vi "SentinelController v33.vi"() -> ()   [LabVIEW 2011] (continued)
                                tunnel: w513 -> [w608]
                                tunnel: w512 -> [w607]
                                frame #0 {
                                n2148 = while {
                                stop <- w517 continue-if-true
                                n2149 = local read "H1 Lock"() -> (w517:bool)
                                n2150 = Wait (ms)(milliseconds to wait=u32 1) -> ()  [unwired: 1 out]
                                }
                                }
                                frame #1 {
                                n2151 = local read "Program Parallelism"() -> (w521:u32)
                                n2152 = local read "H1 parallelism"() -> (w522:u32)
                                n2153 = Less?(x=w522, y=w521) -> (x < y?=w519:bool)
                                n2154 = local read "H1 allow lower parallelism"() -> (w520:bool)
                                n2155 = And(x=w519, y=w520) -> (x .and. y?=w518:bool)
                                n2156 = case shown="False" w518 {
                                tunnel: [w524 w535] -> w523
                                frame False {
                                n2157 = local read "VISA bus 1 resource name out hid"() -> (w532:refnum<visa-resource-name>)
                                n2158 = local read "Binning string from tester hid"() -> (w524:string)
                                n2159 = local read "VISA bus 1 error out hid"() -> (w533:errorcluster)
                                n2160 = local read "GPIB bus 1 traffic"() -> (w528:string)
                                n2161 = VISA Write(VISA resource name=w532, write buffer=w524, error in (no error)=w533) -> (VISA resource name out=w530:refnum<visa-resource-name>, error out=w531:errorcluster)  [unwired: 1 out]
                                n2162 = local write "VISA bus 1 resource name out hid"(w530) -> ()
                                n2163 = local write "VISA bus 1 error out hid"(w531) -> ()
                                n2164 = Unbundle By Name(w531) -> ("status"=w529:bool)
                                n2165 = Concatenate Strings(w528, "\r\n", "Bus 1 write: " ("string"), w524) -> (w526:string)
                                n2166 = local write "GPIB bus 1 write error"(w529) -> ()
                                n2167 = local write "GPIB bus 1 traffic"(w526) -> ()
                                }
                                frame True {
                                n2168 = local read "H1 parallelism"() -> (w534:u32)
                                n2169 = local read "Binning string from tester hid"() -> (w536:string)
                                n2170 = local read "VISA bus 1 resource name out hid"() -> (w547:refnum<visa-resource-name>)
                                n2171 = local read "VISA bus 1 error out hid"() -> (w548:errorcluster)
                                n2172 = Multiply(x=w534, y=u32 8) -> (x*y=w538:u32)
                                n2173 = local read "GPIB bus 1 traffic"() -> (w543:string)
                                n2174 = Decrement(x=w538) -> (x-1=w539:u32)
                                n2175 = String Subset(string=w536, length (rest)=w539) -> (substring=w535:string)  [unwired: 1 in]
                                n2176 = VISA Write(VISA resource name=w547, write buffer=w535, error in (no error)=w548) -> (VISA resource name out=w545:refnum<visa-resource-name>, error out=w546:errorcluster)  [unwired: 1 out]
                                n2177 = local write "VISA bus 1 resource name out hid"(w545) -> ()
                                n2178 = local write "VISA bus 1 error out hid"(w546) -> ()
                                n2179 = Unbundle By Name(w546) -> ("status"=w544:bool)
                                n2180 = Concatenate Strings(w543, "\r\n", "Bus 1 write: " ("string"), w535) -> (w541:string)
                                n2181 = local write "GPIB bus 1 traffic"(w541) -> ()
                                n2182 = local write "GPIB bus 1 write error"(w544) -> ()
                                }
                                }
                                }
                                frame #2 {
                                n2183 = local write "H1 Ready with sites"(FALSE ("waiting")) -> ()
                                n2184 = Tick Count (ms)() -> (millisecond timer value=w551:u32)
                                n2185 = Tick Count (ms)() -> (millisecond timer value=w552:u32)
                                n2186 = local write "H1 tt end hidden"(w551) -> ()
                                n2187 = local write "H1 it start hidden"(w552) -> ()
                                n2188 = local write "H1 Indexing"(TRUE ("waiting")) -> ()
                                n2189 = local write "H1 Testing"(FALSE ("waiting")) -> ()
                                }
                                frame #3 {
                                n2190 = local read "H1 tt start hidden"() -> (w561:u32)
                                n2191 = local read "H1 tt end hidden"() -> (w562:u32)
                                n2192 = while {
                                tunnel: [w580] -> w576 mode=indexing
                                shift-right: [w581] -> _
                                shift-left: w557 -> [w583]
                                stop <- w578 stop-if-true
                                n2193 = Match Pattern(string=w583, regular expression=" ") -> (before substring=w580:string, after substring=w581:string, offset past match=w579:i32)  [unwired: 2 out]
                                n2194 = Less Than 0?(x=w579) -> (x < 0?=w578:bool)
                                }
                                n2195 = Subtract(x=w562, y=w561) -> (x-y=w560:u32)
                                n2196 = Divide(x=w560, y=u32 1000) -> (x/y=w558:dbl)
                                n2197 = local write "H1 measured Test Time"(w558) -> ()
                                n2198 = Array Size(array=w576) -> (size(s)=w573:i32)
                                n2199 = Divide(x=w573, y=3) -> (x/y=w575:dbl)
                                n2200 = To Unsigned Byte Integer(number=w575) -> (unsigned 8bit integer=w571:u8)
                                n2201 = local read "H1 SITES? response hid"() -> (w568:string)
                                n2202 = local read "H1 parallelism"() -> (w567:u32)
                                n2203 = Not Equal?(x=w567, y=w571) -> (x != y?=w572:bool)
                                n2204 = for {
                                N: w571 -> [_]
                                tunnel: w576 -> [w606]
                                tunnel: w568 -> [w597]
                                shift-right: [w590] -> w555
                                shift-left: 0 -> [w589]
                                shift-right: [w586] -> w556
                                shift-left: 0 -> [w584]
                                i -> [w587]
                                n2205 = Increment(x=w584) -> (x+1=w585:i32)
                                n2206 = Increment(x=w589) -> (x+1=w588:i32)
                                n2207 = Increment(x=w587) -> (x+1=w605:i32)
                                n2208 = String Subset(string=w597, offset (0)=w587, length (rest)=1 ("length (rest)")) -> (substring=w593:string)
                                n2209 = Multiply(x=3, y=w605) -> (x*y=w599:i32)
                                n2210 = Equal?(x=w593, y="1") -> (x = y?=w591:bool)
                                n2211 = Decrement(x=w599) -> (x-1=w598:i32)
                                n2212 = Select(t=w588, s=w591, f=w589) -> (s? t:f=w590:i32)
                                n2213 = Index Array(array=w606, index=w598) -> (element=w603:string)
                                n2214 = Decimal String To Number(string=w603, offset=0) -> (number=w601:i32)  [unwired: 1 in, 1 out]
                                n2215 = Equal?(x=w601, y=1) -> (x = y?=w594:bool)
                                n2216 = And(x=w594, y=w591) -> (x .and. y?=w595:bool)
                                n2217 = Select(t=w585, s=w595, f=w584) -> (s? t:f=w586:i32)
                                }
                                n2218 = case shown="True" w572 {
                                frame False {
                                }
                                frame True {
                                n2219 = One Button Dialog(message="Warning:\nH1 Parallelism Mismatch!\nEither allow this from the system configuration tab\nor change the parallelism on H2. This message will\ncontinue until the problem is corrected.") -> ()  [unwired: 1 in, 1 out]
                                }
                                }
                                n2220 = local read "H1 Device Count"() -> (w564:u32)
                                n2221 = local read "H1 Good Units"() -> (w565:u32)
                                n2222 = Add(x=w565, y=w556) -> (x+y=w566:u32)
                                n2223 = Add(x=w564, y=w555) -> (x+y=w563:u32)
                                n2224 = local write "H1 Good Units"(w566) -> ()
                                n2225 = local write "H1 Device Count"(w563) -> ()
                                }
                                frame #4 {
                                n2226 = local read "H1 Device Count"() -> (w612:u32)
                                n2227 = Divide(x=w608, y=w607) -> (x/y=w609:dbl)
                                n2228 = local read "H1 Good Units"() -> (w613:u32)
                                n2229 = Multiply(x=w609, y=100.0) -> (x*y=w611:dbl)
                                n2230 = Divide(x=w613, y=w612) -> (x/y=w616:dbl)
                                n2231 = local write "H1 cycle yield hid"(w611) -> ()
                                n2232 = Multiply(x=w616, y=100.0) -> (x*y=w614:dbl)
                                n2233 = local write "H1 lot yield mon"(w614) -> ()
                                }
                                frame #5 {
                                n2234 = local read "H1 online"() -> (w617:bool)
                                n2235 = local read "POWER"() -> (w618:bool)
                                n2236 = Compound Arithmetic op=AND(w617, w618) -> (w619:bool)
                                n2237 = case shown="True" w619 {
                                frame False {
                                n2238 = local write "MT99XX tester states H1 hid"(SC_MT99XX_tester_states."closing bus" ("SC virtual tester states")) -> ()
                                }
                                frame True {
                                n2239 = local write "MT99XX tester states H1 hid"(SC_MT99XX_tester_states."polling *SITES?" ("SC virtual tester states")) -> ()
                                }
                                }
                                }
                                }
                                }
                                frame "closing bus" {
                                n2240 = local read "GPIB bus 1 traffic"() -> (w626:string)
                                n2241 = local write "Exit SC tester H1 StMach hid"(TRUE ("Exit H1 state machine hid")) -> ()
                                n2242 = local read "VISA bus 1 resource name out hid"() -> (w630:refnum<visa-resource-name>)
                                n2243 = local read "VISA bus 1 error out hid"() -> (w629:errorcluster)
                                n2244 = Concatenate Strings(w626, "\r\n", "Bus 1: closing " ("string")) -> (w624:string)
                                n2245 = local write "GPIB bus 1 traffic"(w624) -> ()
                                n2246 = VISA Close(VISA resource name=w630, error in (no error)=w629) -> (error out=w628:errorcluster)
                                n2247 = Unbundle By Name(w628) -> ("status"=w627:bool)
                                n2248 = local write "VISA bus 1 close error"(w627) -> ()
                                }
                              }
                            }
                            frame #1 {
                              n2249 = local read "Slow for  Diagnostics"() -> (w631:bool)
                              n2250 = case shown="False" w631 {
                                frame False {
                                }
                                frame True {
                                n2251 = local read "GPIB wait time (ms)"() -> (w632:u32)
                                n2252 = Wait (ms)(milliseconds to wait=w632) -> ()  [unwired: 1 out]
                                }
                              }
                            }
                          }
                        }
                        frame "DeltaDesign" {
                          n2253 = local write "MT99XX tester states H1 hid"(SC_MT99XX_tester_states."initializing bus" ("SC virtual tester states")) -> ()
                          n2254 = flat-sequence {
                            frame #0 {
                              n2255 = local read "MT99XX tester states H1 hid"() -> (w634:T4)
                              n2256 = case shown="\"binning\"" w634 {
                                frame "initializing bus", Default {
                                n2257 = flat-sequence {
                                frame #0 {
                                # "bus 1"
                                n2258 = local read "GPIB wait timeout hid"() -> (w638:u32)
                                n2259 = local read "SentCtrl talks to handler 1 at"() -> (w639:refnum<visa-resource-name>)
                                n2260 = local read "GPIB wait timeout hid"() -> (w637:u32)
                                n2261 = VISA Open(timeout (0)=w638, VISA resource name=w639) -> (VISA resource name=w636:refnum<visa-resource-name>, error out=w641:errorcluster)  [unwired: 3 in]
                                n2262 = property class="GPIB Instr"(reference=w636, error in=w641, "Timeout"=w637) -> (error out=w635:errorcluster)  [unwired: 1 out]
                                n2263 = local write "VISA bus 1 resource name out hid"(w636) -> ()
                                n2264 = Unbundle By Name(w635) -> ("status"=w640:bool)
                                n2265 = local write "VISA bus 1 open error"(w640) -> ()
                                n2266 = local write "VISA bus 1 error out hid"(w635) -> ()
                                }
                                frame #1 {
                                n2267 = local write "Exit SC tester H1 StMach hid"(FALSE ("Exit H1 state machine hid")) -> ()
                                n2268 = Concatenate Strings("Bus 1 initializing" ("string"), "\r\n") -> (w644:string)
                                n2269 = local write "GPIB bus 1 traffic"(w644) -> ()
                                }
                                frame #2 {
                                n2270 = local write "MT99XX tester states H1 hid"(SC_MT99XX_tester_states."sending *IDN?" ("SC virtual tester states")) -> ()
                                }
                                }
                                }
                                frame "sending *IDN?" {
                                n2271 = flat-sequence {
                                tunnel: [w656] -> w649
                                tunnel: [w655] -> w648
                                tunnel: w649 -> [w670]
                                tunnel: w648 -> [w669]
                                tunnel: [w660] -> w647
                                tunnel: w647 -> [w671]
                                frame #0 {
                                w650 = "*IDN?"
                                n2272 = local read "VISA bus 1 resource name out hid"() -> (w659:refnum<visa-resource-name>)
                                n2273 = local read "GPIB bus 1 traffic"() -> (w654:string)
                                n2274 = local read "VISA bus 1 error out hid"() -> (w658:errorcluster)
                                n2275 = Concatenate Strings(w654, "\r\n", "Bus 1 write: " ("string"), w650) -> (w652:string)
                                n2276 = VISA Write(VISA resource name=w659, write buffer=w650, error in (no error)=w658) -> (VISA resource name out=w656:refnum<visa-resource-name>, error out=w655:errorcluster)  [unwired: 1 out]
                                n2277 = Unbundle By Name(w655) -> ("status"=w657:bool)
                                n2278 = local write "GPIB bus 1 traffic"(w652) -> ()
                                n2279 = local write "GPIB bus 1 write error"(w657) -> ()
                                }
                                frame #1 {
                                n2280 = local read "GPIB bus 1 traffic"() -> (w662:string)
                                n2281 = VISA Read(VISA resource name=w670, byte count=u32 256, error in (no error)=w669) -> (VISA resource name out=w667:refnum<visa-resource-name>, read buffer=w661:string, error out=w666:errorcluster)  [unwired: 1 out]
                                n2282 = local write "VISA bus 1 resource name out hid"(w667) -> ()
                                n2283 = Unbundle By Name(w666) -> ("status"=w660:bool)
                                n2284 = local write "H1 response to *IDN? hid"(w661) -> ()
                                n2285 = local write "GPIB bus 1 read error"(w660) -> ()
                                n2286 = Concatenate Strings(w662, "\r\n", "Bus 1 read: " ("string"), w661) -> (w664:string)
                                n2287 = local write "GPIB bus 1 traffic"(w664) -> ()
                                }
                                frame #2 {
                                n2288 = case shown="False" w671 {
                                frame False {
                                n2289 = local write "MT99XX tester states H1 hid"(SC_MT99XX_tester_states."polling *SITES?" ("SC virtual tester states")) -> ()
                                }
                                frame True {
                                n2290 = flat-sequence {
                                frame #0 {
                                n2291 = while {
                                stop <- w674 stop-if-true
                                n2292 = One Button Dialog(message="Warning:\nVirtual tester does not get a response\nto *IDN? from handler 1.\nCheck GPIB cable and that  handler 1 \nis running and ready to issue a start of test\nby responding with sites ready.", button name ("OK")="Dismiss and retry") -> (true=w674:bool)
                                n2293 = Wait (ms)(milliseconds to wait=u32 100) -> ()  [unwired: 1 out]
                                }
                                }
                                frame #1 {
                                n2294 = local write "H1 online"(FALSE ("H1 online")) -> ()
                                }
                                frame #2 {
                                n2295 = local write "MT99XX tester states H1 hid"(SC_MT99XX_tester_states."sending *IDN?" ("SC virtual tester states")) -> ()
                                }
                                }
                                }
                                }
                                }
                                }
                                }
                                frame "polling *SITES?" {
                                n2296 = flat-sequence {
                                tunnel: [w682] -> w680
                                tunnel: [w681] -> w679
                                tunnel: w680 -> [w718]
                                tunnel: w679 -> [w717]
                                frame #0 {
                                n2297 = while {
                                tunnel: [w686] -> w682
                                tunnel: [w684] -> w681
                                stop <- w683 stop-if-true
                                n2298 = stacked-sequence {
                                tunnel: [w698] -> w688
                                tunnel: [w697] -> w687
                                frame #0 {
                                w690 = "*SITES?"
                                n2299 = local read "VISA bus 1 resource name out hid"() -> (w696:refnum<visa-resource-name>)
                                n2300 = local read "VISA bus 1 error out hid"() -> (w695:errorcluster)
                                n2301 = Concatenate Strings("Handler 1 cycle start" ("string"), "\r\n", "Bus 1 write: " ("string"), w690) -> (w692:string)
                                n2302 = VISA Write(VISA resource name=w696, write buffer=w690, error in (no error)=w695) -> (VISA resource name out=w698:refnum<visa-resource-name>, error out=w697:errorcluster)  [unwired: 1 out]
                                n2303 = Unbundle By Name(w697) -> ("status"=w694:bool)
                                n2304 = local write "GPIB bus 1 traffic"(w692) -> ()
                                n2305 = local write "GPIB bus 1 write error"(w694) -> ()
                                }
                                }
                                n2306 = Wait (ms)(milliseconds to wait=u32 1) -> ()  [unwired: 1 out]
                                n2307 = flat-sequence {
                                tunnel: w688 -> [w716]
                                tunnel: w687 -> [w715]
                                tunnel: [w703] -> w686
                                tunnel: [w699] -> w684
                                tunnel: [w700] -> w683
                                frame #0 {
                                n2308 = local read "GPIB bus 1 traffic"() -> (w708:string)
                                n2309 = VISA Read(VISA resource name=w716, byte count=u32 256, error in (no error)=w715) -> (read buffer=w703:string, error out=w702:errorcluster)  [unwired: 2 out]
                                n2310 = Unbundle By Name(w702) -> ("status"=w699:bool)
                                n2311 = String Length(string=w703) -> (length=w705:i32)
                                n2312 = Scan Value(string=w703, format string="%b", default (0 dbl)=u8 0) -> (value=w707:u8)  [unwired: 1 out]
                                n2313 = Concatenate Strings(w708, "\r\n", "Bus 1 read: " ("string"), w703) -> (w710:string)
                                n2314 = local write "GPIB bus 1 read error"(w699) -> ()
                                n2315 = Greater Than 0?(x=w705) -> (x > 0?=w704:bool)
                                n2316 = Greater Than 0?(x=w707) -> (x > 0?=w706:bool)
                                n2317 = local write "GPIB bus 1 traffic"(w710) -> ()
                                n2318 = And(x=w704, y=w706) -> (x .and. y?=w701:bool)
                                n2319 = Or(x=w701, y=w699) -> (x .or. y?=w700:bool)
                                }
                                }
                                }
                                }
                                frame #1 {
                                n2320 = case shown="False" w717 {
                                tunnel: w718 -> [w719 _]
                                frame False {
                                n2321 = flat-sequence {
                                tunnel: w719 -> [w720]
                                frame #0 {
                                n2322 = String Length(string=w720) -> (length=w721:i32)
                                n2323 = local write "H1 SITES? response hid"(w720) -> ()
                                n2324 = local write "H1 parallelism"(w721) -> ()
                                }
                                frame #1 {
                                # "This block adds zeroes (sites not ready)\nto SITES READY from handlers when the\nhandler is running at a lower parallelism\nthan the test program, but has the same\npin mapping for the active sites in common."
                                n2325 = local read "Program Parallelism"() -> (w725:u32)
                                n2326 = local read "H1 allow lower parallelism"() -> (w724:bool)
                                n2327 = local read "H1 parallelism"() -> (w726:u32)
                                n2328 = Less?(x=w726, y=w725) -> (x < y?=w723:bool)
                                n2329 = And(x=w723, y=w724) -> (x .and. y?=w722:bool)
                                n2330 = case shown="True" w722 {
                                frame False {
                                n2331 = local read "Program Parallelism"() -> (w729:u32)
                                n2332 = local read "H1 parallelism"() -> (w727:u32)
                                n2333 = Greater?(x=w727, y=w729) -> (0:w728:bool)
                                n2334 = case shown="True" w728 {
                                frame False {
                                # "parallelisms must match if arriving here"
                                n2335 = local write "MT99XX tester states H1 hid"(SC_MT99XX_tester_states."testing" ("SC virtual tester states")) -> ()
                                }
                                frame True {
                                n2336 = local write "MT99XX tester states H1 hid"(SC_MT99XX_tester_states."closing bus" ("SC virtual tester states")) -> ()
                                n2337 = local write "POWER"(FALSE ("POWER")) -> ()
                                n2338 = One Button Dialog(message="Fatal error 300:\nTest program cannot support higher\nparallelism on handler 1.\nThe Sentinel Controller program is shutting down.\nPlease correct the mismatch and restart.") -> ()  [unwired: 1 in, 1 out]
                                }
                                }
                                }
                                frame True {
                                n2339 = local read "Program Parallelism"() -> (w739:u32)
                                n2340 = local read "H1 parallelism"() -> (w736:u32)
                                n2341 = local read "H1 SITES? response hid"() -> (w737:string)
                                n2342 = Subtract(x=w739, y=w736) -> (x-y=w738:u32)
                                n2343 = for {
                                N: w738 -> [_]
                                shift-right: [w740] -> w734
                                shift-left: w737 -> [w741]
                                n2344 = Concatenate Strings(w741, "0" ("string")) -> (w740:string)
                                }
                                n2345 = local write "H1 SITES? response hid"(w734) -> ()
                                n2346 = local write "MT99XX tester states H1 hid"(SC_MT99XX_tester_states."testing" ("SC virtual tester states")) -> ()
                                }
                                }
                                }
                                frame #2 {
                                n2347 = Tick Count (ms)() -> (millisecond timer value=w747:u32)
                                n2348 = Tick Count (ms)() -> (millisecond timer value=w746:u32)
                                n2349 = local write "H1 Ready with sites"(TRUE ("H2 Waiting")) -> ()
                                n2350 = local write "H1 wt start hidden"(w747) -> ()
                                n2351 = local write "H1 it end hidden"(w746) -> ()
                                n2352 = local write "H1 Indexing"(FALSE ("h1 indexing")) -> ()
                                n2353 = local write "H1 Testing"(FALSE ("h1 indexing")) -> ()
                                }
                                frame #3 {
                                n2354 = local read "H1 it start hidden"() -> (w751:u32)
                                n2355 = local read "H1 it end hidden"() -> (w752:u32)
                                n2356 = Subtract(x=w752, y=w751) -> (x-y=w748:u32)
                                n2357 = Divide(x=w748, y=u32 1000) -> (x/y=w750:dbl)
                                n2358 = local write "MT99XX tester states H1 hid"(SC_MT99XX_tester_states."testing" ("SC virtual tester states")) -> ()
                                n2359 = local write "H1 measured Index Time"(w750) -> ()
                                }
                                }
                                }
                                frame True {
                                n2360 = flat-sequence {
                                frame #0 {
                                n2361 = local read "VISA bus 1 resource name out hid"() -> (w756:refnum<visa-resource-name>)
                                n2362 = local read "VISA bus 1 error out hid"() -> (w757:errorcluster)
                                n2363 = VISA Close(VISA resource name=w756, error in (no error)=w757) -> (error out=w755:errorcluster)
                                n2364 = Unbundle By Name(w755) -> ("status"=w754:bool)
                                n2365 = local write "VISA bus 1 close error"(w754) -> ()
                                }
                                frame #1 {
                                n2366 = local write "VISA bus 1 close error"(FALSE ("VISA bus 1 close error")) -> ()
                                n2367 = Concatenate Strings("Bus 1 error  while reading,\nclosing Bus 1 and re-initializing" ("string"), "\r\n") -> (w760:string)
                                n2368 = local write "GPIB bus 1 traffic"(w760) -> ()
                                }
                                frame #2 {
                                n2369 = local write "MT99XX tester states H1 hid"(SC_MT99XX_tester_states."initializing bus" ("SC virtual tester states")) -> ()
                                }
                                }
                                }
                                }
                                }
                                }
                                }
                                frame "testing" {
                                n2370 = flat-sequence {
                                frame #0 {
                                n2371 = while {
                                stop <- w763 stop-if-true
                                n2372 = local read "H1 Lock"() -> (w763:bool)
                                n2373 = Wait (ms)(milliseconds to wait=u32 1) -> ()  [unwired: 1 out]
                                }
                                }
                                frame #1 {
                                n2374 = Tick Count (ms)() -> (millisecond timer value=w774:u32)
                                n2375 = Tick Count (ms)() -> (millisecond timer value=w773:u32)
                                n2376 = local write "H1 Testing"(TRUE ("testing")) -> ()
                                n2377 = local write "H1 Ready with sites"(FALSE ("H1 Waiting")) -> ()
                                n2378 = local write "H1 Indexing"(FALSE ("waiting")) -> ()
                                n2379 = local write "H1 wt end hidden"(w774) -> ()
                                n2380 = local write "H1 tt start hidden"(w773) -> ()
                                n2381 = local read "GPIB bus 1 traffic"() -> (w766:string)
                                n2382 = Concatenate Strings(w766, "\r\n", "Bus 1: " ("string"), "testing" ("string")) -> (w768:string)
                                n2383 = local write "GPIB bus 1 traffic"(w768) -> ()
                                }
                                frame #2 {
                                n2384 = local read "H1 wt start hidden"() -> (w778:u32)
                                n2385 = local read "H1 wt end hidden"() -> (w779:u32)
                                n2386 = Subtract(x=w779, y=w778) -> (x-y=w777:u32)
                                n2387 = Divide(x=w777, y=u32 1000) -> (x/y=w775:dbl)
                                n2388 = local write "H1 measured Wait Time"(w775) -> ()
                                }
                                frame #3 {
                                n2389 = local write "MT99XX tester states H1 hid"(SC_MT99XX_tester_states."binning" ("SC virtual tester states")) -> ()
                                }
                                }
                                }
                                frame "binning" {
                                n2390 = flat-sequence {
                                tunnel: [w792] -> w784
                                tunnel: [w819] -> w783
                                tunnel: w784 -> [w819]
                                tunnel: w783 -> [w826]
                                tunnel: [w825] -> w782
                                tunnel: [w824] -> w781
                                tunnel: w782 -> [w877]
                                tunnel: w781 -> [w876]
                                frame #0 {
                                n2391 = while {
                                stop <- w786 continue-if-true
                                n2392 = local read "H1 Lock"() -> (w786:bool)
                                n2393 = Wait (ms)(milliseconds to wait=u32 1) -> ()  [unwired: 1 out]
                                }
                                }
                                frame #1 {
                                n2394 = local read "Program Parallelism"() -> (w790:u32)
                                n2395 = local read "H1 parallelism"() -> (w791:u32)
                                n2396 = Less?(x=w791, y=w790) -> (x < y?=w788:bool)
                                n2397 = local read "H1 allow lower parallelism"() -> (w789:bool)
                                n2398 = And(x=w788, y=w789) -> (x .and. y?=w787:bool)
                                n2399 = case shown="False" w787 {
                                tunnel: [w793 w804] -> w792
                                frame False {
                                n2400 = local read "VISA bus 1 resource name out hid"() -> (w801:refnum<visa-resource-name>)
                                n2401 = local read "Binning string from tester hid"() -> (w793:string)
                                n2402 = local read "VISA bus 1 error out hid"() -> (w802:errorcluster)
                                n2403 = local read "GPIB bus 1 traffic"() -> (w797:string)
                                n2404 = VISA Write(VISA resource name=w801, write buffer=w793, error in (no error)=w802) -> (VISA resource name out=w799:refnum<visa-resource-name>, error out=w800:errorcluster)  [unwired: 1 out]
                                n2405 = local write "VISA bus 1 resource name out hid"(w799) -> ()
                                n2406 = local write "VISA bus 1 error out hid"(w800) -> ()
                                n2407 = Unbundle By Name(w800) -> ("status"=w798:bool)
                                n2408 = Concatenate Strings(w797, "\r\n", "Bus 1 write: " ("string"), w793) -> (w795:string)
                                n2409 = local write "GPIB bus 1 write error"(w798) -> ()
                                n2410 = local write "GPIB bus 1 traffic"(w795) -> ()
                                }
                                frame True {
                                n2411 = local read "H1 parallelism"() -> (w803:u32)
                                n2412 = local read "Binning string from tester hid"() -> (w805:string)
                                n2413 = local read "VISA bus 1 resource name out hid"() -> (w816:refnum<visa-resource-name>)
                                n2414 = local read "VISA bus 1 error out hid"() -> (w817:errorcluster)
                                n2415 = Multiply(x=w803, y=u32 8) -> (x*y=w807:u32)
                                n2416 = local read "GPIB bus 1 traffic"() -> (w812:string)
                                n2417 = Decrement(x=w807) -> (x-1=w808:u32)
                                n2418 = String Subset(string=w805, length (rest)=w808) -> (substring=w804:string)  [unwired: 1 in]
                                n2419 = VISA Write(VISA resource name=w816, write buffer=w804, error in (no error)=w817) -> (VISA resource name out=w814:refnum<visa-resource-name>, error out=w815:errorcluster)  [unwired: 1 out]
                                n2420 = local write "VISA bus 1 resource name out hid"(w814) -> ()
                                n2421 = local write "VISA bus 1 error out hid"(w815) -> ()
                                n2422 = Unbundle By Name(w815) -> ("status"=w813:bool)
                                n2423 = Concatenate Strings(w812, "\r\n", "Bus 1 write: " ("string"), w804) -> (w810:string)
                                n2424 = local write "GPIB bus 1 traffic"(w810) -> ()
                                n2425 = local write "GPIB bus 1 write error"(w813) -> ()
                                }
                                }
                                }
                                frame #2 {
                                n2426 = local write "H1 Ready with sites"(FALSE ("waiting")) -> ()
                                n2427 = Tick Count (ms)() -> (millisecond timer value=w820:u32)
                                n2428 = Tick Count (ms)() -> (millisecond timer value=w821:u32)
                                n2429 = local write "H1 tt end hidden"(w820) -> ()
                                n2430 = local write "H1 it start hidden"(w821) -> ()
                                n2431 = local write "H1 Indexing"(TRUE ("waiting")) -> ()
                                n2432 = local write "H1 Testing"(FALSE ("waiting")) -> ()
                                }
                                frame #3 {
                                n2433 = local read "H1 tt start hidden"() -> (w830:u32)
                                n2434 = while {
                                tunnel: [w849] -> w845 mode=indexing
                                shift-right: [w850] -> _
                                shift-left: w826 -> [w852]
                                stop <- w847 stop-if-true
                                n2435 = Match Pattern(string=w852, regular expression=" ") -> (before substring=w849:string, after substring=w850:string, offset past match=w848:i32)  [unwired: 2 out]
                                n2436 = Less Than 0?(x=w848) -> (x < 0?=w847:bool)
                                }
                                n2437 = local read "H1 tt end hidden"() -> (w831:u32)
                                n2438 = Subtract(x=w831, y=w830) -> (x-y=w829:u32)
                                n2439 = Divide(x=w829, y=u32 1000) -> (x/y=w827:dbl)
                                n2440 = local write "H1 measured Test Time"(w827) -> ()
                                n2441 = Array Size(array=w845) -> (size(s)=w842:i32)
                                n2442 = Divide(x=w842, y=3) -> (x/y=w844:dbl)
                                n2443 = To Unsigned Byte Integer(number=w844) -> (unsigned 8bit integer=w840:u8)
                                n2444 = local read "H1 SITES? response hid"() -> (w837:string)
                                n2445 = local read "H1 parallelism"() -> (w836:u32)
                                n2446 = Not Equal?(x=w836, y=w840) -> (x != y?=w841:bool)
                                n2447 = for {
                                N: w840 -> [_]
                                tunnel: w845 -> [w875]
                                tunnel: w837 -> [w866]
                                shift-right: [w859] -> w824
                                shift-left: 0 -> [w858]
                                shift-right: [w855] -> w825
                                shift-left: 0 -> [w853]
                                i -> [w856]
                                n2448 = Increment(x=w853) -> (x+1=w854:i32)
                                n2449 = Increment(x=w858) -> (x+1=w857:i32)
                                n2450 = Increment(x=w856) -> (x+1=w874:i32)
                                n2451 = String Subset(string=w866, offset (0)=w856, length (rest)=1 ("length (rest)")) -> (substring=w862:string)
                                n2452 = Multiply(x=3, y=w874) -> (x*y=w868:i32)
                                n2453 = Equal?(x=w862, y="1") -> (x = y?=w860:bool)
                                n2454 = Decrement(x=w868) -> (x-1=w867:i32)
                                n2455 = Select(t=w857, s=w860, f=w858) -> (s? t:f=w859:i32)
                                n2456 = Index Array(array=w875, index=w867) -> (element=w872:string)
                                n2457 = Decimal String To Number(string=w872, offset=0) -> (number=w870:i32)  [unwired: 1 in, 1 out]
                                n2458 = Equal?(x=w870, y=1) -> (x = y?=w863:bool)
                                n2459 = And(x=w863, y=w860) -> (x .and. y?=w864:bool)
                                n2460 = Select(t=w854, s=w864, f=w853) -> (s? t:f=w855:i32)
                                }
                                n2461 = case shown="True" w841 {
                                frame False {
                                }
                                frame True {
                                n2462 = One Button Dialog(message="Warning:\nH1 Parallelism Mismatch!\nEither allow this from the system configuration tab\nor change the parallelism on H2. This message will\ncontinue until the problem is corrected.") -> ()  [unwired: 1 in, 1 out]
                                }
                                }
                                n2463 = local read "H1 Device Count"() -> (w833:u32)
                                n2464 = local read "H1 Good Units"() -> (w834:u32)
                                n2465 = Add(x=w834, y=w825) -> (x+y=w835:u32)
                                n2466 = Add(x=w833, y=w824) -> (x+y=w832:u32)
                                n2467 = local write "H1 Good Units"(w835) -> ()
                                n2468 = local write "H1 Device Count"(w832) -> ()
                                }
                                frame #4 {
                                n2469 = local read "H1 Device Count"() -> (w881:u32)
                                n2470 = Divide(x=w877, y=w876) -> (x/y=w878:dbl)
                                n2471 = local read "H1 Good Units"() -> (w882:u32)
                                n2472 = Multiply(x=w878, y=100.0) -> (x*y=w880:dbl)
                                n2473 = Divide(x=w882, y=w881) -> (x/y=w885:dbl)
                                n2474 = local write "H1 cycle yield hid"(w880) -> ()
                                n2475 = Multiply(x=w885, y=100.0) -> (x*y=w883:dbl)
                                n2476 = local write "H1 lot yield mon"(w883) -> ()
                                }
                                frame #5 {
                                n2477 = local read "H1 online"() -> (w886:bool)
                                n2478 = local read "POWER"() -> (w887:bool)
                                n2479 = Compound Arithmetic op=AND(w886, w887) -> (w888:bool)
                                n2480 = case shown="True" w888 {
                                frame False {
                                n2481 = local write "MT99XX tester states H1 hid"(SC_MT99XX_tester_states."closing bus" ("SC virtual tester states")) -> ()
                                }
                                frame True {
                                n2482 = local write "MT99XX tester states H1 hid"(SC_MT99XX_tester_states."polling *SITES?" ("SC virtual tester states")) -> ()
                                }
                                }
                                }
                                }
                                }
                                frame "closing bus" {
                                n2483 = local read "GPIB bus 1 traffic"() -> (w895:string)
                                n2484 = local write "Exit SC tester H1 StMach hid"(TRUE ("Exit H1 state machine hid")) -> ()
                                n2485 = local read "VISA bus 1 resource name out hid"() -> (w899:refnum<visa-resource-name>)
                                n2486 = local read "VISA bus 1 error out hid"() -> (w898:errorcluster)
                                n2487 = Concatenate Strings(w895, "\r\n", "Bus 1: closing " ("string")) -> (w893:string)
                                n2488 = local write "GPIB bus 1 traffic"(w893) -> ()
                                n2489 = VISA Close(VISA resource name=w899, error in (no error)=w898) -> (error out=w897:errorcluster)
                                n2490 = Unbundle By Name(w897) -> ("status"=w896:bool)
                                n2491 = local write "VISA bus 1 close error"(w896) -> ()
                                }
                              }
                            }
                            frame #1 {
                              n2492 = local read "Slow for  Diagnostics"() -> (w900:bool)
                              n2493 = case shown="False" w900 {
                                frame False {
                                }
                                frame True {
                                n2494 = local read "GPIB wait time (ms)"() -> (w901:u32)
                                n2495 = Wait (ms)(milliseconds to wait=w901) -> ()  [unwired: 1 out]
                                }
                              }
                            }
                          }
                        }
                        frame "Seiko-Epson NS6040" {
                          n2496 = local write "NS6040 tester states H1 hid"(SC_NS6040_tester_states."initializing bus" ("NS6040 tester states H1 hid")) -> ()
                          n2497 = while {
                            stop <- w903 stop-if-true
                            n2498 = flat-sequence {
                              frame #0 {
                                n2499 = local read "NS6040 tester states H1 hid"() -> (w904:T3)
                                n2500 = case shown="\"testing\"" w904 {
                                frame "initializing bus", Default {
                                n2501 = flat-sequence {
                                frame #0 {
                                # "bus 1"
                                n2502 = local read "GPIB wait timeout hid"() -> (w908:u32)
                                n2503 = local read "SentCtrl talks to handler 1 at"() -> (w909:refnum<visa-resource-name>)
                                n2504 = local read "GPIB wait timeout hid"() -> (w907:u32)
                                n2505 = VISA Open(timeout (0)=w908, VISA resource name=w909) -> (VISA resource name=w906:refnum<visa-resource-name>, error out=w911:errorcluster)  [unwired: 3 in]
                                n2506 = property class="GPIB Instr"(reference=w906, error in=w911, "Timeout"=w907) -> (error out=w905:errorcluster)  [unwired: 1 out]
                                n2507 = local write "VISA bus 1 resource name out hid"(w906) -> ()
                                n2508 = Unbundle By Name(w905) -> ("status"=w910:bool)
                                n2509 = local write "VISA bus 1 open error"(w910) -> ()
                                n2510 = local write "VISA bus 1 error out hid"(w905) -> ()
                                }
                                frame #1 {
                                n2511 = local write "Exit SC tester H1 StMach hid"(FALSE ("Exit H1 state machine hid")) -> ()
                                n2512 = Concatenate Strings("Bus 1 initializing" ("string"), "\r\n") -> (w914:string)
                                n2513 = local write "GPIB bus 1 traffic"(w914) -> ()
                                }
                                frame #2 {
                                n2514 = local write "NS6040 tester states H1 hid"(SC_NS6040_tester_states."serial polling handler" ("NS6040 tester states H1 hid")) -> ()
                                }
                                }
                                }
                                frame "sending *IDN?" {
                                n2515 = flat-sequence {
                                tunnel: [w926] -> w919
                                tunnel: [w925] -> w918
                                tunnel: w919 -> [w940]
                                tunnel: w918 -> [w939]
                                tunnel: [w930] -> w917
                                tunnel: w917 -> [w941]
                                frame #0 {
                                w920 = "*IDN?\n"
                                # "It was discovered that his state is not initialized in application"
                                n2516 = local read "VISA bus 1 resource name out hid"() -> (w929:refnum<visa-resource-name>)
                                n2517 = local read "GPIB bus 1 traffic"() -> (w924:string)
                                n2518 = local read "VISA bus 1 error out hid"() -> (w928:errorcluster)
                                n2519 = Concatenate Strings(w924, "\r\n", "Bus 1 write: " ("string"), w920) -> (w922:string)
                                n2520 = VISA Write(VISA resource name=w929, write buffer=w920, error in (no error)=w928) -> (VISA resource name out=w926:refnum<visa-resource-name>, error out=w925:errorcluster)  [unwired: 1 out]
                                n2521 = Unbundle By Name(w925) -> ("status"=w927:bool)
                                n2522 = local write "GPIB bus 1 traffic"(w922) -> ()
                                n2523 = local write "GPIB bus 1 write error"(w927) -> ()
                                }
                                frame #1 {
                                n2524 = local read "GPIB bus 1 traffic"() -> (w932:string)
                                n2525 = VISA Read(VISA resource name=w940, byte count=u32 256, error in (no error)=w939) -> (VISA resource name out=w937:refnum<visa-resource-name>, read buffer=w931:string, error out=w936:errorcluster)  [unwired: 1 out]
                                n2526 = local write "VISA bus 1 resource name out hid"(w937) -> ()
                                n2527 = Unbundle By Name(w936) -> ("status"=w930:bool)
                                n2528 = local write "H1 response to *IDN? hid"(w931) -> ()
                                n2529 = local write "GPIB bus 1 read error"(w930) -> ()
                                n2530 = Concatenate Strings(w932, "\r\n", "Bus 1 read: " ("string"), w931) -> (w934:string)
                                n2531 = local write "GPIB bus 1 traffic"(w934) -> ()
                                }
                                frame #2 {
                                n2532 = case shown="False" w941 {
                                frame False {
                                n2533 = local write "NS6040 tester states H1 hid"(SC_NS6040_tester_states."sending SRQ MASK" ("NS6040 tester states H1 hid")) -> ()
                                }
                                frame True {
                                n2534 = flat-sequence {
                                frame #0 {
                                n2535 = while {
                                stop <- w944 stop-if-true
                                n2536 = One Button Dialog(message="Warning:\nVirtual tester does not get a response\nto *IDN? from handler 1.\nCheck GPIB cable and that  handler 1 \nis running and ready to issue a start of test\nby responding with sites ready.", button name ("OK")="Dismiss and retry") -> (true=w944:bool)
                                n2537 = Wait (ms)(milliseconds to wait=u32 100) -> ()  [unwired: 1 out]
                                }
                                }
                                frame #1 {
                                n2538 = local write "H1 online"(FALSE ("H1 online")) -> ()
                                }
                                frame #2 {
                                n2539 = local write "NS6040 tester states H1 hid"(SC_NS6040_tester_states."sending *IDN?" ("NS6040 tester states H1 hid")) -> ()
                                }
                                }
                                }
                                }
                                }
                                }
                                }
                                frame "sending SRQ MASK" {
                                n2540 = flat-sequence {
                                tunnel: [w950] -> w949
                                tunnel: w949 -> [w959]
                                frame #0 {
                                w951 = "SRQ MASK 65\n"
                                # "It was discovered that his state is not initialized in application"
                                n2541 = local read "VISA bus 1 resource name out hid"() -> (w958:refnum<visa-resource-name>)
                                n2542 = local read "VISA bus 1 error out hid"() -> (w957:errorcluster)
                                n2543 = local read "GPIB bus 1 traffic"() -> (w955:string)
                                n2544 = VISA Write(VISA resource name=w958, write buffer=w951, error in (no error)=w957) -> (error out=w956:errorcluster)  [unwired: 2 out]
                                n2545 = Unbundle By Name(w956) -> ("status"=w950:bool)
                                n2546 = Concatenate Strings(w955, "\r\n", "Bus 1 write: " ("string"), w951) -> (w953:string)
                                n2547 = local write "GPIB bus 1 traffic"(w953) -> ()
                                n2548 = local write "GPIB bus 1 write error"(w950) -> ()
                                }
                                frame #1 {
                                n2549 = case shown="False" w959 {
                                frame False {
                                n2550 = local write "NS6040 tester states H1 hid"(SC_NS6040_tester_states."serial polling handler" ("NS6040 tester states H1 hid")) -> ()
                                }
                                frame True {
                                n2551 = flat-sequence {
                                frame #0 {
                                n2552 = while {
                                stop <- w962 stop-if-true
                                n2553 = Wait (ms)(milliseconds to wait=u32 100) -> ()  [unwired: 1 out]
                                n2554 = One Button Dialog(message="Error when writing SRQ MASK to handler 1.\nClosing bus 1.", button name ("OK")="Dismiss and retry") -> (true=w962:bool)
                                }
                                }
                                frame #1 {
                                n2555 = local write "H1 online"(FALSE ("H1 online")) -> ()
                                }
                                frame #2 {
                                n2556 = local write "NS6040 tester states H1 hid"(SC_NS6040_tester_states."closing bus" ("NS6040 tester states H1 hid")) -> ()
                                }
                                }
                                }
                                }
                                }
                                }
                                }
                                frame "serial polling handler" {
                                w968 = "1"
                                w982 = "%08b"  # format string
                                n2557 = flat-sequence {
                                tunnel: [w989] -> w983
                                tunnel: [w988] -> _
                                frame #0 {
                                n2558 = local read "VISA bus 1 resource name out hid"() -> (w992:refnum<visa-resource-name>)
                                n2559 = local read "VISA bus 1 error out hid"() -> (w991:errorcluster)
                                n2560 = local write "GPIB bus 1 traffic"("Serial polling handler 1") -> ()
                                n2561 = VISA Read STB(8:w991, 11:w992) -> (0:w993:errorcluster, 2:w989:u16)  [unwired: 1 out]
                                n2562 = Unbundle By Name(w993) -> ("status"=w988:bool)
                                n2563 = local write "GPIB bus 1 write error"(w988) -> ()
                                }
                                }
                                n2564 = Format Into String "Format Into String"(format string=w982, w983) -> (resulting string=w969:string)  [unwired: 2 in, 1 out]
                                n2565 = local read "GPIB bus 1 traffic"() -> (w981:string)
                                n2566 = String Subset(string=w969, offset (0)=1, length (rest)=1 ("length (rest)")) -> (substring=w974:string)
                                n2567 = String Subset(string=w969, offset (0)=7, length (rest)=1 ("length (rest)")) -> (substring=w975:string)
                                n2568 = Equal?(x=w974, y=w968) -> (x = y?=w973:bool)
                                n2569 = Equal?(x=w968, y=w975) -> (x = y?=w972:bool)
                                n2570 = Concatenate Strings(w981, "\r\n", "Bus 1 read: " ("string"), w969) -> (w979:string)
                                n2571 = And(x=w973, y=w972) -> (x .and. y?=w967:bool)
                                n2572 = case shown="True" w967 {
                                frame False {
                                n2573 = flat-sequence {
                                frame #0 {
                                n2574 = Wait (ms)(milliseconds to wait=u32 5) -> ()  [unwired: 1 out]
                                }
                                frame #1 {
                                n2575 = local write "NS6040 tester states H1 hid"(SC_NS6040_tester_states."serial polling handler" ("NS6040 tester states H1 hid")) -> ()
                                }
                                }
                                }
                                frame True {
                                # "This is where the GPIB0 bus controller (PXI Chassis, instrument) has its STB set to 0100 0001 which signals to the tester that a handler is ready with sites"
                                n2576 = flat-sequence {
                                frame #0 {
                                n2577 = local write "H1 Ready with sites"(TRUE ("H1 Ready with sites")) -> ()
                                }
                                frame #1 {
                                n2578 = local write "NS6040 tester states H1 hid"(SC_NS6040_tester_states."sending Fullsites?" ("NS6040 tester states H1 hid")) -> ()
                                }
                                }
                                }
                                }
                                n2579 = local write "GPIB bus 1 traffic"(w979) -> ()
                                }
                                frame "sending FR? " {
                                n2580 = while {
                                tunnel: [w995] -> w994
                                stop <- w998 stop-if-true
                                n2581 = Wait (ms)(milliseconds to wait=u32 20) -> ()  [unwired: 1 out]
                                n2582 = flat-sequence {
                                tunnel: [w1008] -> w1002
                                tunnel: [w1007] -> w1001
                                tunnel: w1002 -> [w1012]
                                tunnel: w1001 -> [w1011]
                                tunnel: [w1010] -> w995
                                tunnel: [w1009] -> w997
                                frame #0 {
                                w1003 = "FR?"
                                # "It was discovered that his state is not initialized in application"
                                n2583 = local read "VISA bus 1 resource name out hid"() -> (w1006:refnum<visa-resource-name>)
                                n2584 = local read "VISA bus 1 error out hid"() -> (w1005:errorcluster)
                                n2585 = local write "GPIB bus 1 traffic"(w1003) -> ()
                                n2586 = VISA Write(VISA resource name=w1006, write buffer=w1003, error in (no error)=w1005) -> (VISA resource name out=w1008:refnum<visa-resource-name>, error out=w1007:errorcluster)  [unwired: 1 out]
                                n2587 = Unbundle By Name(w1007) -> ("status"=w1004:bool)
                                n2588 = local write "GPIB bus 1 write error"(w1004) -> ()
                                }
                                frame #1 {
                                n2589 = local read "GPIB bus 1 traffic"() -> (w1019:string)
                                n2590 = VISA Read(VISA resource name=w1012, byte count=u32 4096, error in (no error)=w1011) -> (VISA resource name out=w1014:refnum<visa-resource-name>, read buffer=w1009:string, error out=w1015:errorcluster)  [unwired: 1 out]
                                n2591 = local write "VISA bus 1 resource name out hid"(w1014) -> ()
                                n2592 = local write "H1 response to FR? hid"(w1009) -> ()
                                n2593 = Unbundle By Name(w1015) -> ("status"=w1010:bool)
                                n2594 = local write "GPIB bus 1 read error"(w1010) -> ()
                                n2595 = Concatenate Strings(w1019, "\r\n", "Bus 1 read: " ("string"), w1009) -> (w1017:string)
                                n2596 = local write "GPIB bus 1 traffic"(w1017) -> ()
                                }
                                }
                                n2597 = Equal?(x=w997, y="FR0") -> (x = y?=w1000:bool)
                                n2598 = Or(x=w1000, y=w995) -> (x .or. y?=w998:bool)
                                }
                                n2599 = case shown="False" w994 {
                                frame False {
